vi "Example 2 - Read.vi"() -> ()   [LabVIEW 2021]
uses:
  SharedVariable_Bus/SharedVariable_Bus.lvclass
  C:/Program Files (x86)/National Instruments/LabVIEW 2021/vi.lib/TSA/Omni-Bus/Omni-Bus/Bus Access/Bus_Access.lvclass
  <vilib>/TSA/Omni-Bus/Omni-Bus/Omni_Bus.lvclass
  <vilib>/TSA/Omni-Bus/Omni-Bus/Support/Read/Read Boolean.vi
  <vilib>/TSA/Omni-Bus/Omni-Bus/Support/Read/Read DBL.vi
  <vilib>/TSA/Omni-Bus/Omni-Bus/Support/Write/Write Boolean.vi
  <vilib>/TSA/Omni-Bus/Omni-Bus/Support/Write/Write DBL.vi
  <vilib>/TSA/Abstract Data Classes/Abs_Types/Boolean/Abs_Boolean.lvclass
  <vilib>/TSA/Abstract Data Classes/Abs_Types/Double Float/Abs_Double Float.lvclass
panel:
  out "Numeric 2":dbl
  out "Boolean 2":bool
  in  "stop":bool
  in  "Numeric":dbl
  in  "Boolean":bool
  out "DBL":dbl
  out "Bool":bool
  out "Tags":string[](array[string])
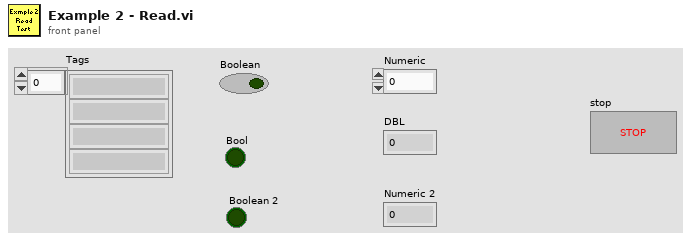
[diagram p1: front panel]
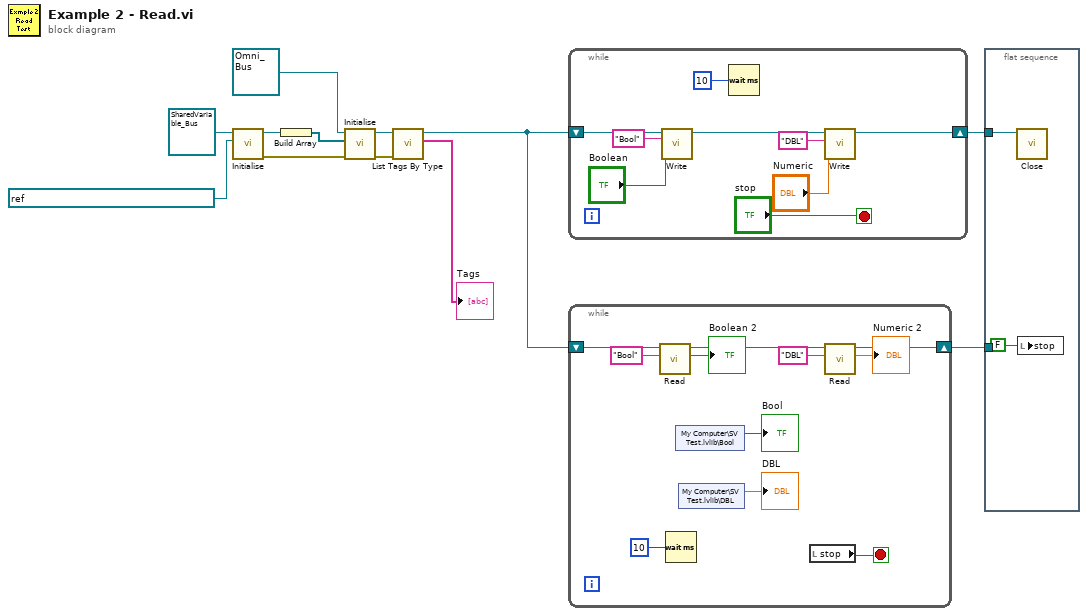
[diagram p0: block diagram]
diagram:
  n1 = call "Initialise.vi"("SV Container"=refnum<k21> "ni.var.psp://my computer/SV Test" ("container refnum in"), "SharedVariable_Bus in"=refnum<class "SharedVariable_Bus.lvclass"> refnum) -> ("error out"=w10:errorcluster, "SharedVariable_Bus out"=w9:refnum<class "SharedVariable_Bus.lvclass">)  [unwired: 8 in]
  n2 = Build Array(w9) -> (w8:refnum<class "SharedVariable_Bus.lvclass">[])
  n3 = call-dynamic "Initialise.vi"("error in (no error)"=w10, "Bus Access"=w8, "Var Bus in"=refnum<class "Omni_Bus.lvclass"> refnum) -> ("error out"=w5:errorcluster, "Var Bus out"=w6:refnum<class "Omni_Bus.lvclass">)  [unwired: 7 in]
  n4 = call-dynamic "List Tags By Type.vi"("error in (no error)"=w5, "Var Bus in"=w6) -> ("Tags"=→"Tags":string[], "Var Bus out"=w2:refnum<class "Omni_Bus.lvclass">)  [unwired: 6 in, 2 out]
  n5 = while {
    shift-right: [w19] -> w3
    shift-left: w2 -> [w21]
    stop <- "stop" stop-if-true
    n6 = call-poly <vilib>:"Write.vi"("Boolean"="Boolean", "Tag"="Bool", "Omni_Bus in"=w21) -> ("Omni_Bus out"=w20:refnum<class "Omni_Bus.lvclass">)  [unwired: 7 in, 1 out]
    n7 = Wait (ms)(milliseconds to wait=u32 10) -> ()  [unwired: 1 out]
    n8 = call-poly <vilib>:"Write.vi"("Numeric"="Numeric", "Tag"="DBL", "Omni_Bus in"=w20) -> ("Omni_Bus out"=w19:refnum<class "Omni_Bus.lvclass">)  [unwired: 7 in, 1 out]
  }
  n9 = while {
    shift-right: [w24] -> w1
    shift-left: w2 -> [w28]
    stop <- w30 stop-if-true
    n10 = call-poly <vilib>:"Read.vi"("Tag"="Bool", "Var Bus in"=w28) -> ("Boolean"=→"Boolean 2":bool, "Var Bus out"=w25:refnum<class "Omni_Bus.lvclass">)  [unwired: 7 in, 1 out]
    n11 = Wait (ms)(milliseconds to wait=u32 10) -> ()  [unwired: 1 out]
    n12 = shared-variable "My Computer\\SV Test.lvlib\\Bool"() -> (→"Bool":bool)  [unwired: 1 in, 1 out]
    n13 = shared-variable "My Computer\\SV Test.lvlib\\DBL"() -> (→"DBL":dbl)  [unwired: 1 in, 1 out]
    n14 = local read "stop"() -> (w30:bool)
    n15 = call-poly <vilib>:"Read.vi"("Tag"="DBL", "Var Bus in"=w25) -> ("Numeric"=→"Numeric 2":dbl, "Var Bus out"=w24:refnum<class "Omni_Bus.lvclass">)  [unwired: 7 in, 1 out]
  }
  n16 = flat-sequence {
    tunnel: w3 -> [w34]
    tunnel: w1 -> [_]
    frame #0 {
      n17 = call-dynamic "Close.vi"("Data in"=w34) -> ()  [unwired: 9 in, 2 out]
      n18 = local write "stop"(FALSE ("stop")) -> ()
    }
  }
